vi "Get Approved and Recieved Paths.vi"(10 "This VI":path) -> (1 "Recieved":path, 2 "Approved Path":path)   [LabVIEW 2020, in "Basic Mechanics Tests.lvclass"]
uses:
  Basic Mechanics Tests.lvclass
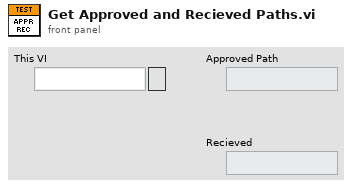
[diagram p1: front panel]
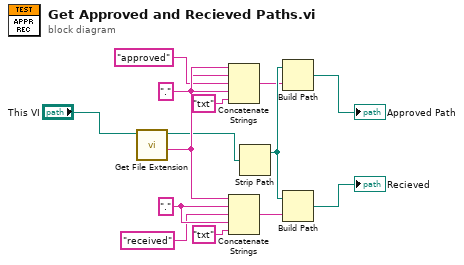
[diagram p0: block diagram]
diagram:
  w8 = "." ("string")
  w3 = "." ("string")
  n1 = call <vilib>:"Get File Extension.vi"("file"="This VI") -> ("filename without extension"=w9:string, "dup file"=w2:path)  [unwired: 6 in, 3 out]
  n2 = Concatenate Strings(w9, w3, "approved" ("string"), w3, "txt" ("string")) -> (w5:string)
  n3 = Concatenate Strings(w9, w8, "received" ("string"), w8, "txt" ("string")) -> (w6:string)
  n4 = Strip Path(path=w2) -> (stripped path=w10:path)  [unwired: 1 out]
  n5 = Build Path(base path=w10, name or relative path=w5) -> (appended path=→"Approved Path":path)
  n6 = Build Path(base path=w10, name or relative path=w6) -> (appended path=→"Recieved":path)
